vi "ModelCutPlaneIntersect.vi"(10 "CuttingZ":sgl, 11 "Triangles":T3[](array[typedef])) -> (2 "NumTriIntersected":i32, 3 "LineArray":T1[](array[typedef]))   [LabVIEW 2014]
uses:
  TypeDefs/TriangleFace.ctl
  TypeDefs/Point3D.ctl
  TypeDefs/Line2D.ctl
  TypeDefs/Point2DwSlope.ctl
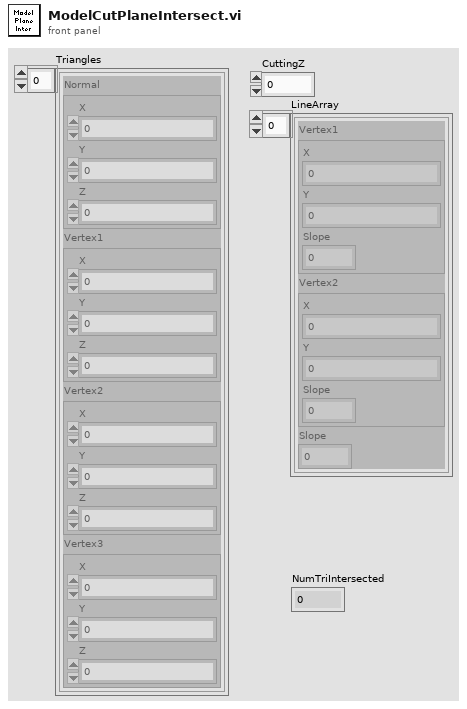
[diagram p1: front panel]
types:
  T1 = typedef "Line2D.ctl" = cluster{"Vertex1":T2, "Vertex2":T2, "Slope":dbl}
  T2 = typedef "Point2DwSlope.ctl" = cluster{"X":sgl, "Y":sgl, "Slope":dbl}
  T3 = typedef "TriangleFace.ctl" = cluster{"Normal":T4, "Vertex1":T4, "Vertex2":T4, "Vertex3":T4}
  T4 = typedef "Point3D.ctl" = cluster{"X":sgl, "Y":sgl, "Z":sgl}
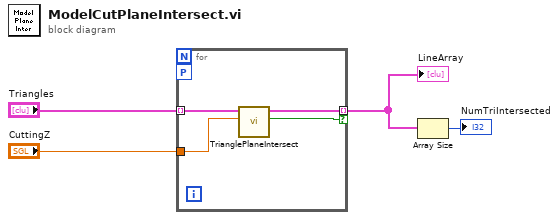
[diagram p0: block diagram]
diagram:
  n1 = for {
    tunnel: "Triangles" -> [w8] mode=indexing
    workers-P: _ -> [_]
    tunnel: "CuttingZ" -> [w7]
    tunnel: [w6] -> w2 mode=indexing if=w5
    n2 = call "TrianglePlaneIntersect.vi"("CuttingZ"=w7, "TriangleFace"=w8) -> ("Intersects?"=w5:bool, "Line2D"=w6:T1)  [unwired: 8 in]
  }
  "LineArray" <- w2
  n3 = Array Size(array=w2) -> (size(s)=→"NumTriIntersected":i32)
